vi "Get Channel Values.vi"(7 "Time in Step":dbl, 8 "error in (no error)":errorcluster, 9 "Default Value":dbl, 10 "Previous Value":dbl, 11 "Channel Value Expression":T1) -> (0 "error out":errorcluster, 3 "Channel Values":dbl[](array[numeric]))   [LabVIEW 2020, in "Output Sequencer.lvlib" / "Output Sequencer.lvclass"]
uses:
  Output Sequencer.lvclass
  Types/Expression Data.ctl
  <vilib>/LAVA/muParser/mupExpr/mupExpr.lvclass
  <vilib>/LAVA/muParser/mupExpr/mupExpr.lvclass/mupExpr.ctl
  <vilib>/LAVA/muParser/mupExpr/Eval_MultiVar_MultiRes.vi
  <vilib>/LAVA/muParser/mupExpr/SetVarVal.vi
  <vilib>/LAVA/muParser/mupLib/mupEvalMulti.vi
  <vilib>/LAVA/muParser/mupLib/mupSetVarValue.vi
  <vilib>/LAVA/muParser/mupLib/mupCheckError.vi
  <vilib>/Utility/error.llb/Error Cluster From Error Code.vi
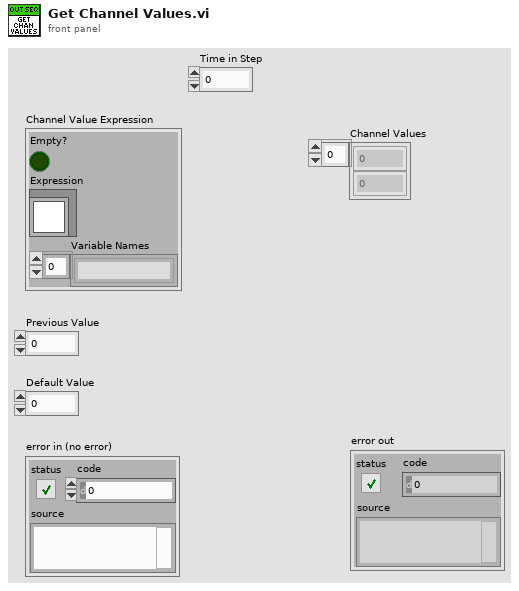
[diagram p1: front panel]
types:
  T1 = typedef "Output Sequencer.lvlib/Output Sequencer.lvclass/Expression Data.ctl" = cluster{"Empty?":bool, "Expression":refnum<class "mupExpr.lvclass">, "Variable Names":string[]}
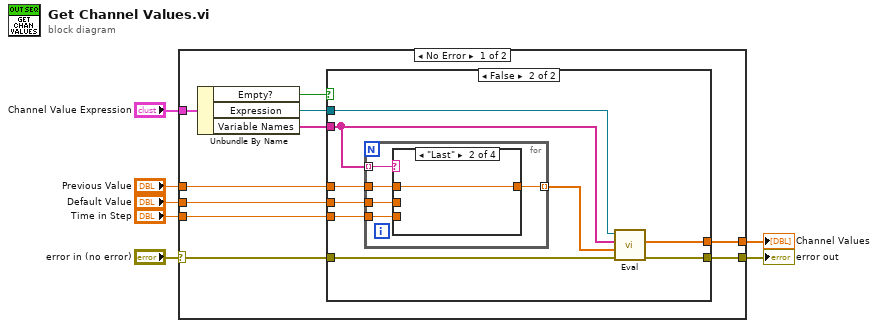
[diagram p0: block diagram]
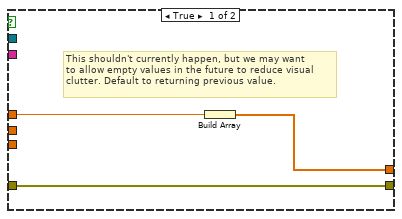
[diagram p2: hidden frame]
diagram:
  n1 = case shown="No Error" "error in (no error)" {
    selector: "error in (no error)" -> [w8 w38]
    tunnel: [w17 _] -> w7
    tunnel: "Previous Value" -> [w16 _]
    tunnel: "Channel Value Expression" -> [w15 _]
    tunnel: "Default Value" -> [w14 _]
    tunnel: "Time in Step" -> [w13 _]
    tunnel: [w9 w38] -> w2
    frame No Error {
      n2 = Unbundle By Name(w15) -> ("Empty?"=w12:bool, "Expression"=w10:refnum<class "mupExpr.lvclass">, "Variable Names"=w11:string[])
      n3 = case shown="False" w12 {
        tunnel: [w20 w29] -> w17
        tunnel: w16 -> [w19 w28]
        tunnel: w14 -> [_ w27]
        tunnel: w13 -> [_ w26]
        tunnel: w11 -> [_ w24]
        tunnel: w10 -> [_ w23]
        tunnel: w8 -> [w18 w21]
        tunnel: [w18 w22] -> w9
        frame True {
          # "This shouldn't currently happen, but we may want\nto allow empty values in the future to reduce visual\nclutter. Default to returning previous value."
          n4 = Build Array(w19) -> (w20:dbl[])
        }
        frame False {
          n5 = for {
            tunnel: w24 -> [w34] mode=indexing
            tunnel: [w33] -> w25 mode=indexing
            tunnel: w28 -> [w32]
            tunnel: w27 -> [w31]
            tunnel: w26 -> [w30]
            n6 = case shown="\"Last\"" w34 {
              tunnel: [_ w35 w36 w37] -> w33
              tunnel: w32 -> [_ w35 _ _]
              tunnel: w31 -> [_ _ w36 _]
              tunnel: w30 -> [_ _ _ w37]
              frame Default {
                # "Shouldn't happen.\nVariables validated\non compile."
              }
              frame "Last" {
              }
              frame "Default" {
              }
              frame "t" {
              }
            }
          }
          n7 = call-poly <vilib>:"Eval.vi"("error in (no error)"=w21, "varValues"=w25, "varNames"=w24, "muExpr in"=w23) -> ("error out"=w22:errorcluster, "Results"=w29:dbl[])  [unwired: 5 in, 1 out]
        }
      }
    }
    frame Error {
    }
  }
  "Channel Values" <- w7
  "error out" <- w2
